vi "acquire one scan.vi"(8 "error in":errorcluster, 11 "taskID in":refnum<k21>) -> (0 "error out":errorcluster, 1 "scans read":u32, 2 "voltage data":dbl[][](array[numeric]) format="%.6f", 3 "taskID out":refnum<k21>, 4 "status":bool)   [LabVIEW 2012]
doc: "Cont(inuous) Acq(uire) & Chart (buffered) demonstrates buffered data acquisition. Data is continuously acquired into a circular buffer at the same time that data previously retrieved from the buffer is plotted. This VI also demonstrates how to plot multiple points from multiple channels on a chart. \n\nBefore running this VI, set the values of the controls on the front panel. Select Show Help Window from the Help menu to see a description of each control. If the values you select for all the controls are values you will usually use, select Make Current Values Default from the Operate menu and save the VI. Or, you may save individual control's default values by popping up on the control, selecting Data Operations, then selecting Make Current Value Default, and saving the VI.\n\n\nThe buffer size is the number of scans that will be held in the internal memory buffer, and is limited by the amount of memory available. In order to keep up with the scan rate as best as possible, this VI retrieves either \"min # of scans to read at a time\" or the scan backlog from the previous AI Read call, whichever is greater. Experiment with the buffer size and the number of scans to read each time. If the buffer is too small or you are not reading data from it fast enough, your data will be overwritten by new data before you have a chance to read it (overwrite error). If the buffer is too big, you will run out of memory (out of memory error).\n\n\nYou will probably want to add more functions to the diagram to customize this VI for your application. A common reason to read data while the acquisition is in progress is to process and display the data in pseudo-real time. The acquisition rate you can achieve depends on how much processing and display the VI must do. This VI calls a subVI named My Data Processing. Add whatever processing you need to this subVI, or replace it with one of your own. The data processing subVI also demonstrates how to use error clusters in your own subVIs, so they can be included in the error data flow chain. Note that the amount of the data returned will change depending on the scan backlog. Use the \"number read\" output from the AI Read VI to determine how many scans are returned."
uses:
  <vilib>/DAQmx/read.llb/DAQmx Read (Analog 2D DBL NChan NSamp).vi
  <vilib>/DAQmx/miscellaneous.llb/DAQmx Fill In Error Info.vi
  <resource>/objmgr/daqmx.rc
panel:
  in  "milliseconds to wait":u32=10
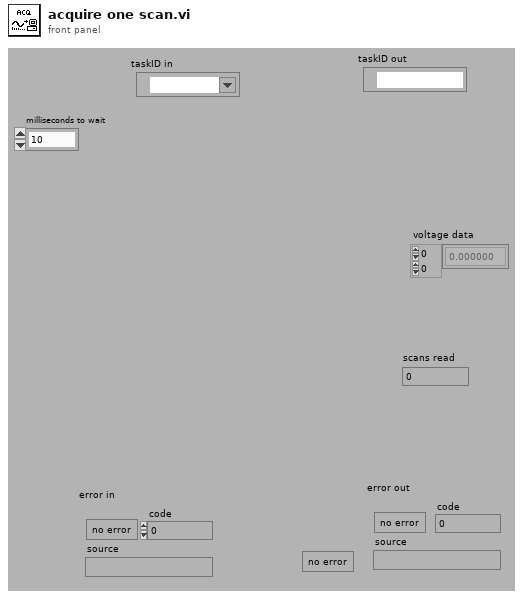
[diagram p1: front panel]
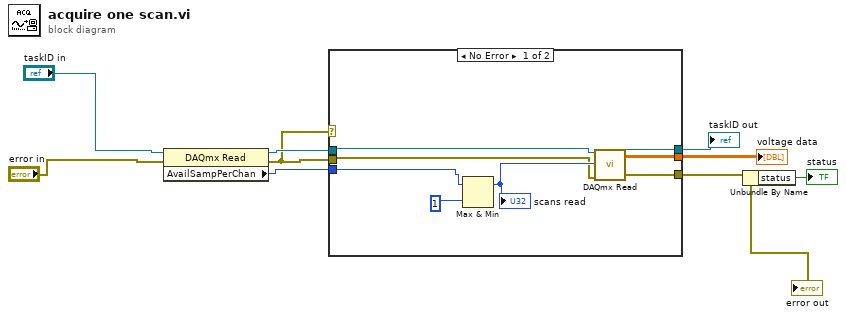
[diagram p0: block diagram]
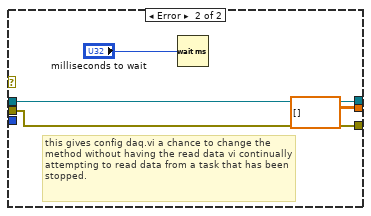
[diagram p2: hidden frame]
diagram:
  n1 = property class="DAQmx Read"(reference="taskID in", error in="error in") -> (reference out=w4:refnum<k21>, error out=w2:errorcluster, "AvailSampPerChan"=w1:u32)
  n2 = case shown="No Error" w2 {
    tunnel: w4 -> [w12 w21]
    tunnel: w2 -> [w11 w20]
    tunnel: [w17 w20] -> w6
    tunnel: [w16 dbl[][] [] ("data")] -> w8
    tunnel: [w15 w21] -> w7
    tunnel: w1 -> [w10 _]
    frame No Error {
      n3 = Max & Min(x=w10, y=1 ("f")) -> (max(x,y)=w13:u32)  [unwired: 1 out]
      "scans read" <- w13
      n4 = call-poly <vilib>:"DAQmx Read.vi"("task/channels in"=w12, "number of samples per channel"=w13, "error in"=w11) -> ("task out"=w15:refnum<k21>, "data"=w16:dbl[][], "error out"=w17:errorcluster)  [unwired: 10 in]
    }
    frame Error {
      # "this gives config daq.vi a chance to change the method without having the read data vi continually attempting to read data from a task that has been stopped."
      n5 = Wait (ms)(milliseconds to wait="milliseconds to wait") -> ()  [unwired: 1 out]
    }
  }
  "taskID out" <- w7
  "error out" <- w6
  "voltage data" <- w8
  n6 = Unbundle By Name(w6) -> ("status"=→"status":bool)
